vi "Generate Digital Lines String.vi"(8 "Numeric":i32=24, 10 "Port":dbl, 11 "Device":dbl) -> (3 "lines":tag)   [LabVIEW 2013]
panel:
  out "String":string
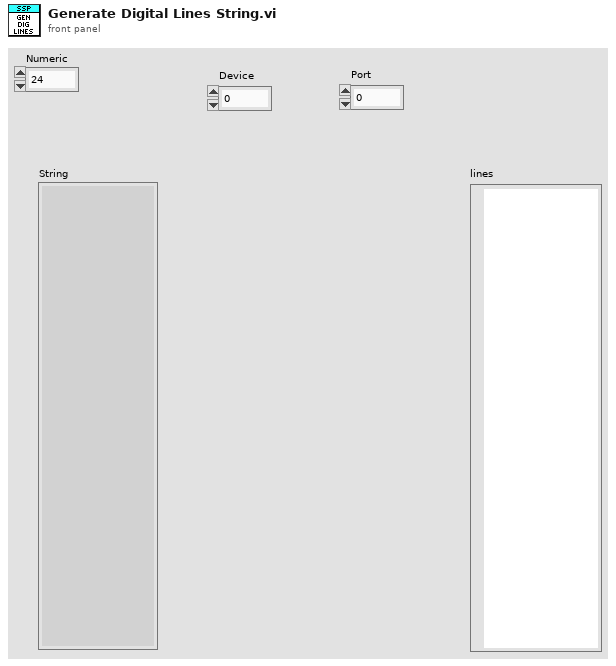
[diagram p1: front panel]
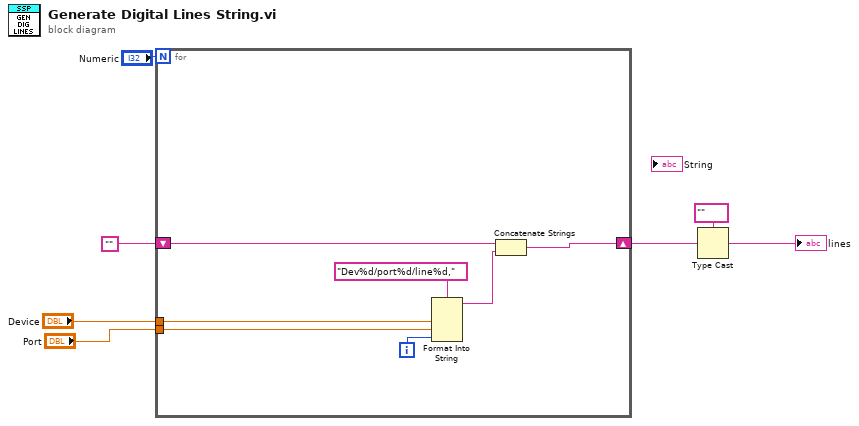
[diagram p0: block diagram]
diagram:
  n1 = for {
    N: "Numeric" -> [_]
    shift-right: [w13] -> w2
    shift-left: "" -> [w14]
    tunnel: "Device" -> [w11]
    tunnel: "Port" -> [w10]
    i -> [w9]
    n2 = Format Into String(format string="Dev%d/port%d/line%d,", w11, w10, w9) -> (resulting string=w8:string)  [unwired: 2 in, 1 out]
    n3 = Concatenate Strings(w14, w8) -> (w13:string)
  }
  n4 = Type Cast(type=tag "" ("*(type *) &x"), x=w2) -> (*(type *) &x=→"lines":tag)
